vi "OP10B_Data.vi"() -> (0 "OP10B_002_SLEEVE_PIN_SEAL_ASSY":T1)   [LabVIEW 2020]
uses:
  Controls/OP10B_DataCluster.ctl
panel:
  out "[SLEEVE_LOAD_MIN]":dbl
  out "[SLEEVE_LOAD]":dbl
  out "[SLEEVE_LOAD_MAX]":dbl
  out "[SLEEVE_HEIGHT_MIN]":dbl
  out "[SLEEVE_HEIGHT]":dbl
  out "[SLEEVE_HEIGHT_MAX]":dbl
  out "[PIN_LOAD_MIN]":dbl
  out "[PIN_LOAD]":dbl
  out "[PIN_LOAD_MAX]":dbl
  out "[PIN_HEIGHT_MIN]":dbl
  out "[PIN_HEIGHT]":dbl
  out "[PIN_HEIGHT_MAX]":dbl
  out "[SEAL_VAC_MIN]":dbl
  out "[SEAL_VAC]":dbl
  out "[SEAL_VAC_MAX]":dbl
  out "[CT]":dbl
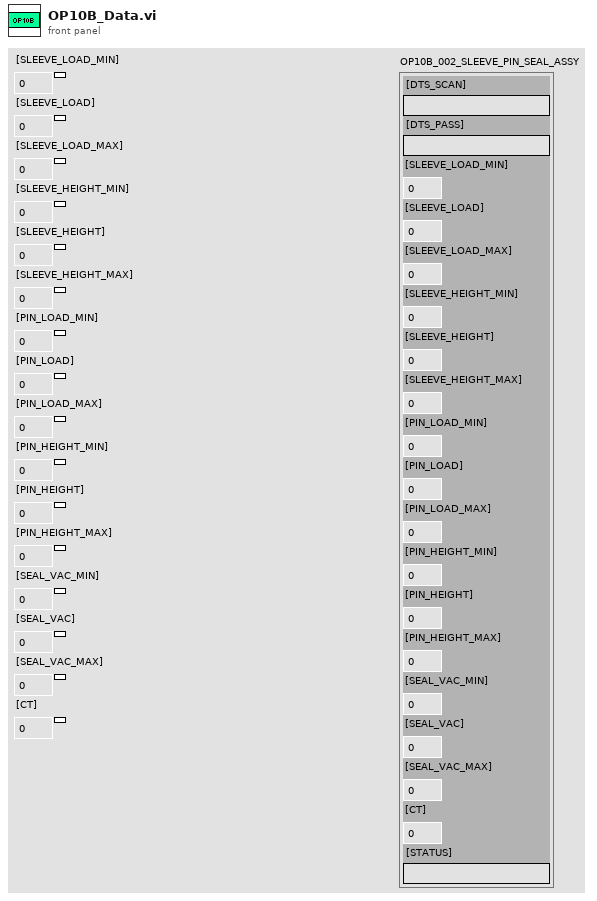
[diagram p1: front panel]
types:
  T1 = typedef "OP10B_DataCluster.ctl" = cluster{"[DTS_SCAN]":string, "[DTS_PASS]":string, "[SLEEVE_LOAD_MIN]":dbl, "[SLEEVE_LOAD]":dbl, "[SLEEVE_LOAD_MAX]":dbl, "[SLEEVE_HEIGHT_MIN]":dbl, "[SLEEVE_HEIGHT]":dbl, "[SLEEVE_HEIGHT_MAX]":dbl, "[PIN_LOAD_MIN]":dbl, "[PIN_LOAD]":dbl, "[PIN_LOAD_MAX]":dbl, "[PIN_HEIGHT_MIN]":dbl, "[PIN_HEIGHT]":dbl, "[PIN_HEIGHT_MAX]":dbl, "[SEAL_VAC_MIN]":dbl, "[SEAL_VAC]":dbl, "[SEAL_VAC_MAX]":dbl, "[CT]":dbl, "[STATUS]":string}
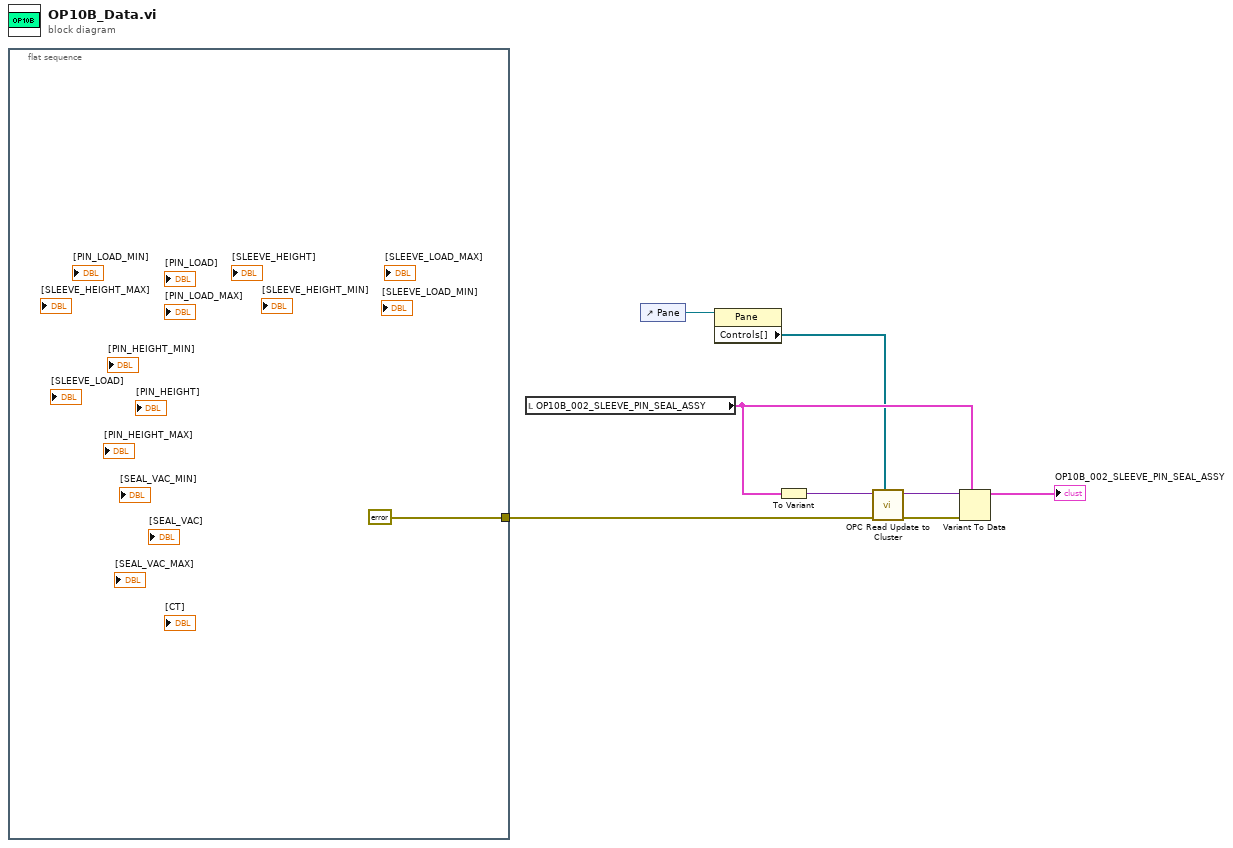
[diagram p0: block diagram]
diagram:
  n1 = flat-sequence {
    tunnel: [errorcluster {"status"=FALSE, "code"=0, "source"=""} ("error in (no error)")] -> w3
    frame #0 {
    }
  }
  n2 = local read "OP10B_002_SLEEVE_PIN_SEAL_ASSY"() -> (w5:T1)
  n3 = control-ref of="Pane"() -> (w2:refnum<vi>)
  n4 = property class="Pane"(reference=w2) -> ("Controls[]"=w1:refnum<vi>[])  [unwired: 1 in, 2 out]
  n5 = To Variant(anything=w5) -> (Variant=w6:variant)
  n6 = call "OPC Read Update to Cluster.vi"("Controls[]"=w1, "error in (no error)"=w3, "Variant in"=w6) -> ("error out"=w7:errorcluster, "Variant out"=w8:variant)  [unwired: 7 in]
  n7 = Variant To Data(error in=w7, type=w5, Variant=w8) -> (data=→"OP10B_002_SLEEVE_PIN_SEAL_ASSY":T1)  [unwired: 1 out]
